vi "Is palindrome-string.vi"(1 "string in":string) -> (0 "T = string is a palindrome":bool)   [LabVIEW 2021, in "Numeric Utilities.lvlib"]
uses:
  Numeric Utilities.lvlib
panel:
  out "Loop iteration":i32
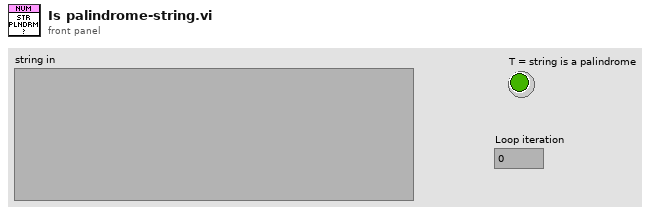
[diagram p1: front panel]
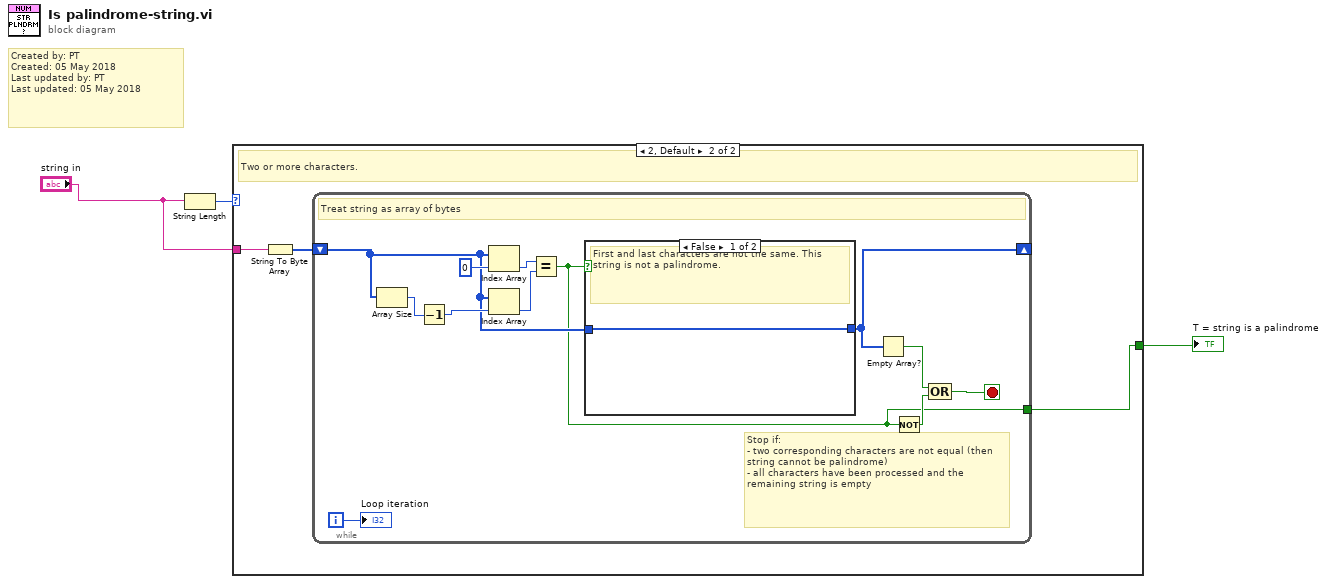
[diagram p0: block diagram]
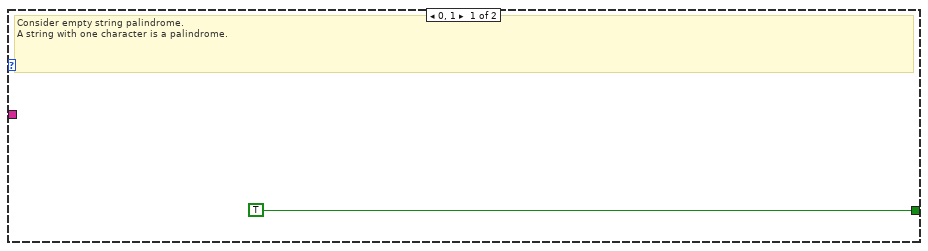
[diagram p2: hidden frame]
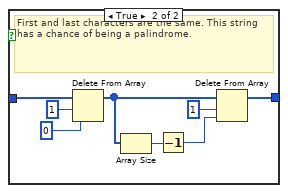
[diagram p3: hidden frame]
diagram:
  # "Created by: PT\nCreated: 05 May 2018\nLast updated by: PT\nLast updated: 05 May 2018"
  n1 = String Length(string="string in") -> (length=w3:i32)
  n2 = case shown="2, Default" w3 {
    tunnel: [TRUE w5] -> w2
    tunnel: "string in" -> [_ w7]
    frame 0, 1 {
      # "Consider empty string palindrome.\nA string with one character is a palindrome."
    }
    frame 2, Default {
      # "Two or more characters."
      n3 = String To Byte Array(string=w7) -> (unsigned byte array=w6:u8[])
      n4 = while {
        shift-right: [w13] -> _
        shift-left: w6 -> [w14]
        tunnel: [w9] -> w5
        i -> [w8]
        stop <- w10 stop-if-true
        # "Stop if:\n- two corresponding characters are not equal (then string cannot be palindrome)\n- all characters have been processed and the remaining string is empty"
        # "Treat string as array of bytes"
        n5 = Array Size(array=w14) -> (size(s)=w19:i32)
        n6 = Decrement(x=w19) -> (x-1=w17:i32)
        n7 = Index Array(array=w14, index=0) -> (element=w16:u8)
        n8 = Index Array(array=w14, index=w17) -> (element=w15:u8)
        n9 = Equal?(x=w16, y=w15) -> (x = y?=w9:bool)
        n10 = case shown="False" w9 {
          tunnel: w14 -> [w20 w28]
          tunnel: [w20 w21] -> w13
          frame False {
            # "First and last characters are not the same. This string is not a palindrome."
          }
          frame True {
            # "First and last characters are the same. This string has a chance of being a palindrome."
            n11 = Delete From Array(array=w28, length=1, index=0) -> (array with subset deleted=w23:u8[])  [unwired: 1 out]
            n12 = Array Size(array=w23) -> (size(s)=w24:i32)
            n13 = Decrement(x=w24) -> (x-1=w22:i32)
            n14 = Delete From Array(array=w23, length=1, index=w22) -> (array with subset deleted=w21:u8[])  [unwired: 1 out]
          }
        }
        n15 = Empty Array?(array=w13) -> (empty?=w12:bool)
        n16 = Not(x=w9) -> (.not. x?=w11:bool)
        n17 = Compound Arithmetic op=OR(w12, w11) -> (w10:bool)
        "Loop iteration" <- w8
      }
    }
  }
  "T = string is a palindrome" <- w2
